vi "MTMount_acceptCommand_abort.vi"(8 "error in (no error)":errorcluster, 11 "command_abort_Ctl":T1) -> (0 "error out":errorcluster, 2 "function return":i32, 3 "command_abort_Ctl out":T1)   [LabVIEW 2018, in "SALLV_MTMount.lvlib"]
doc: "int MTMount_shm_acceptCommand_abortLV(MTMount_command_abortLV *command_abort_Ctl );"
uses:
  SALLV_MTMount.lvlib
  DataTypes/command_abort.ctl
  SALLV_MTMount.so
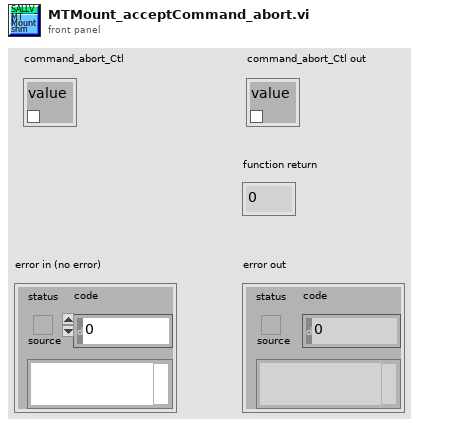
[diagram p1: front panel]
types:
  T1 = typedef "SALLV_MTMount.lvlib/command_abort.ctl" = cluster{"value":bool}
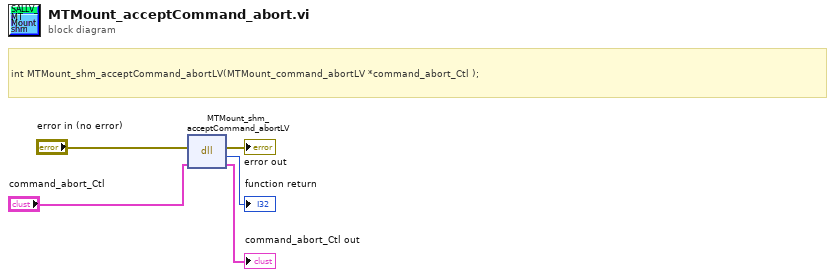
[diagram p0: block diagram]
diagram:
  # "int MTMount_shm_acceptCommand_abortLV(MTMount_command_abortLV *command_abort_Ctl );"
  n1 = dll-call lib="home/ttsai/Document/salApiMTMount/SALLV_MTMount/SALLV_MTMount.*" fn="MTMount_shm_acceptCommand_abortLV"(error in="error in (no error)", "command_abort_Ctl"="command_abort_Ctl") -> (error out=→"error out":errorcluster, →"function return":i32, "command_abort_Ctl"=→"command_abort_Ctl out":T1)  [unwired: 2 in, 1 out]
